vi "Графики-07-wdt.vi"() -> ()   [LabVIEW 2017]
uses:
  <vilib>/measure/NI_MABase.lvlib
panel:
  out "Waveform Graph":dbl[](graph)
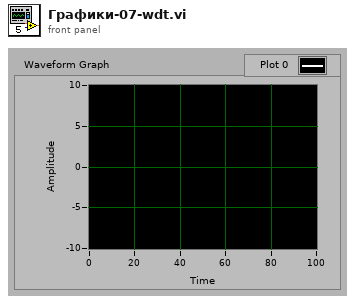
[diagram p1: front panel]
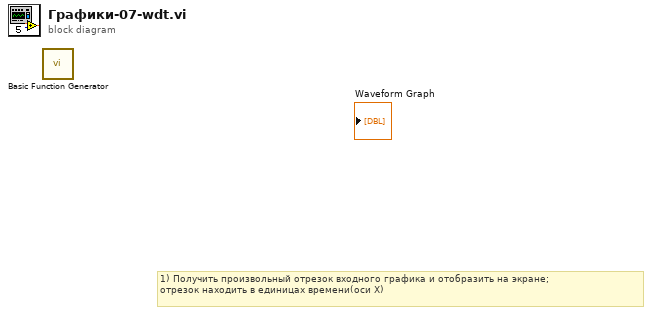
[diagram p0: block diagram]
diagram:
  # "1) Получить произвольный отрезок входного графика и отобразить на экране; \nотрезок находить в единицах времени(оси Х)"
  n1 = call <vilib>:"Basic Function Generator.vi"() -> ()  [unwired: 9 in, 3 out]
